vi "Parse_TCP_Message_From_Unity.vi"(5 "Tokenized message string array":string[](array[string])) -> (2 "task Over Message Received Flag":bool, 3 "Desired tensions by motor":T1, 4 "Control point position coords":dbl[](array[numeric]), 6 "Command string":string, 8 "Force field type specifier":string, 10 "Center point of FF":dbl[](array[numeric]), 13 "File information string":string, 14 "Trunk Structure Matrix":dbl[][](array[numeric]), 15 "Boundary points":dbl[](array[numeric]))   [LabVIEW 2024]
panel:
  out "Corresponding motor tensions":dbl[](array[numeric])
  out "Motor numbers":i32[](array[numeric])
  out "Most Recent Vicon Frame Number":u32
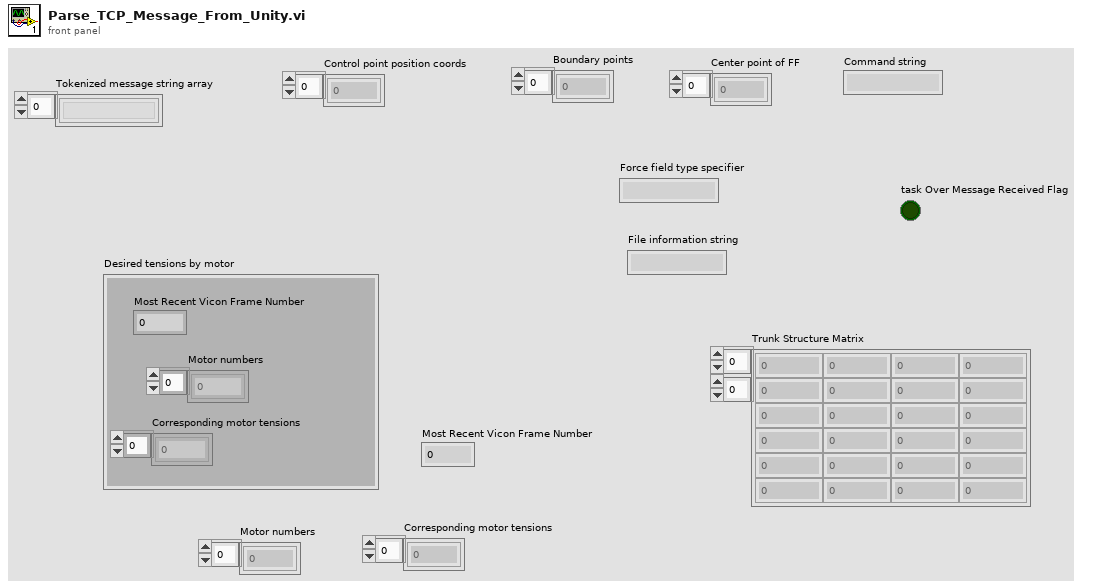
[diagram p1: front panel]
types:
  T1 = cluster{"Most Recent Vicon Frame Number":u32, "Corresponding motor tensions":dbl[], "Motor numbers":i32[]}
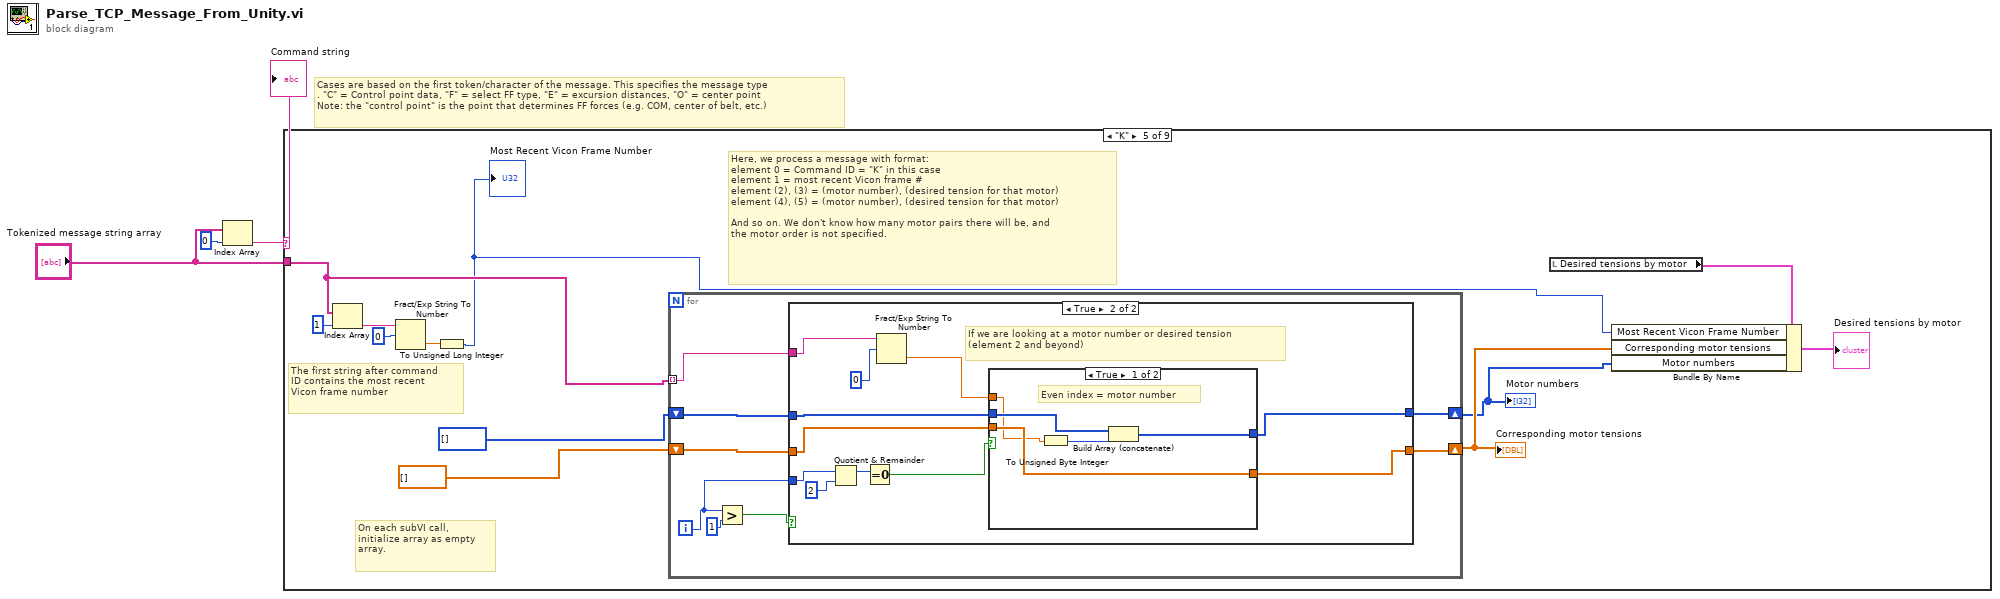
[diagram p0: block diagram]
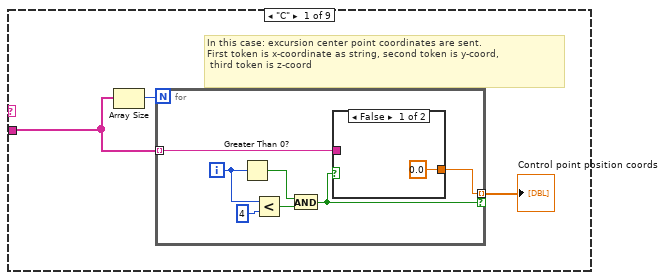
[diagram p2: hidden frame]
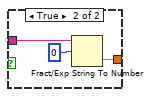
[diagram p3: hidden frame]
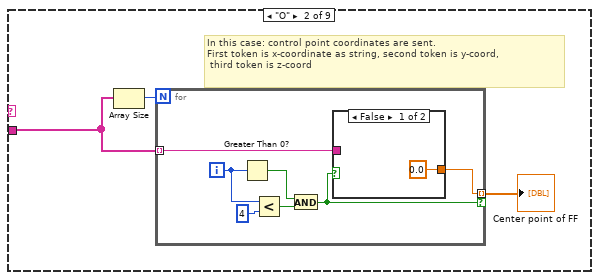
[diagram p4: hidden frame]
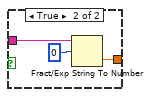
[diagram p5: hidden frame]
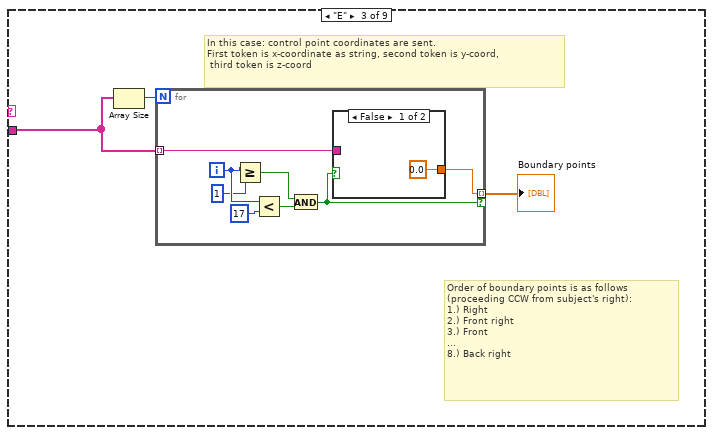
[diagram p6: hidden frame]
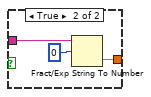
[diagram p7: hidden frame]
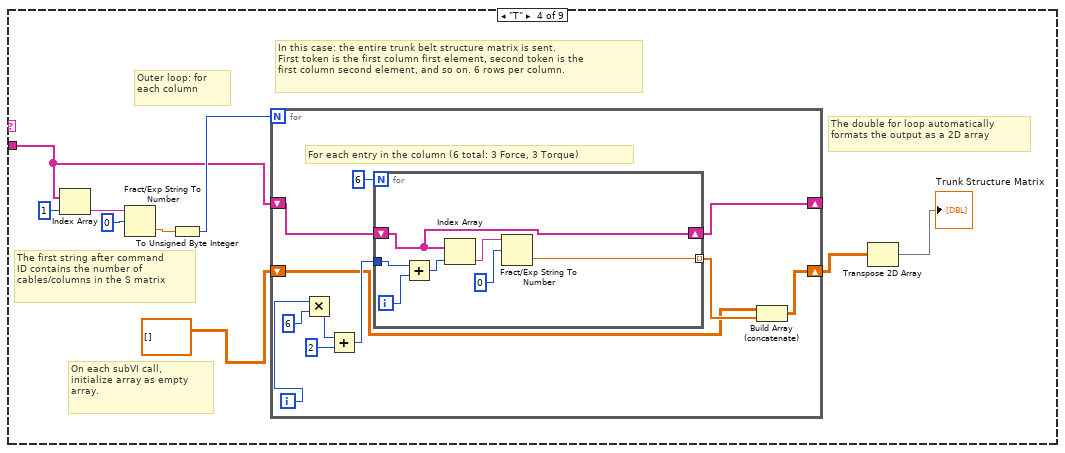
[diagram p8: hidden frame]
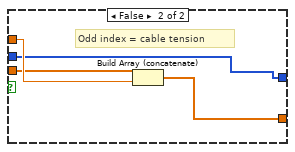
[diagram p10: hidden frame]
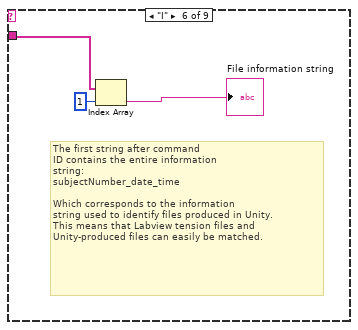
[diagram p11: hidden frame]
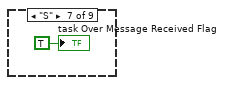
[diagram p12: hidden frame]
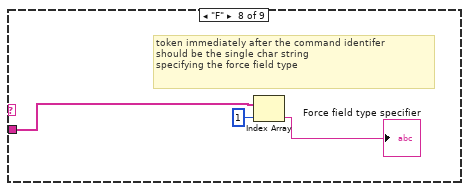
[diagram p13: hidden frame]
diagram:
  # "Cases are based on the first token/character of the message. This specifies the message type\n. \"C\" = Control point data, \"F\" = select FF type, \"E\" = excursion distances, \"O\" = center point \nNote: the \"control point\" is the point that determines FF forces (e.g. COM, center of belt, etc.)"
  n1 = Index Array(array="Tokenized message string array", index=0) -> (element=w2:string)
  "Command string" <- w2
  n2 = case shown="\"K\"" w2 {
    tunnel: "Tokenized message string array" -> [w4 w18 w32 w50 w82 w117 _ w121 _]
    frame "C" {
      # "In this case: excursion center point coordinates are sent. \nFirst token is x-coordinate as string, second token is y-coord,\n third token is z-coord"
      n3 = Array Size(array=w4) -> (size(s)=w6:i32)
      n4 = for {
        N: w6 -> [_]
        tunnel: w4 -> [w13] mode=indexing
        tunnel: [w12] -> w5 mode=indexing if=w7
        i -> [w9]
        n5 = Greater Than 0?(x=w9) -> (x > 0?=w11:bool)
        n6 = Less?(x=w9, y=4) -> (x < y?=w10:bool)
        n7 = And(x=w11, y=w10) -> (x .and. y?=w7:bool)
        n8 = case shown="False" w7 {
          tunnel: w13 -> [_ w17]
          tunnel: [0.0 w15] -> w12
          frame False {
          }
          frame True {
            n9 = Fract/Exp String To Number(string=w17, offset=0) -> (number=w15:dbl)  [unwired: 2 in, 1 out]
          }
        }
      }
      "Control point position coords" <- w5
    }
    frame "O" {
      # "In this case: control point coordinates are sent. \nFirst token is x-coordinate as string, second token is y-coord,\n third token is z-coord"
      n10 = Array Size(array=w18) -> (size(s)=w20:i32)
      n11 = for {
        N: w20 -> [_]
        tunnel: w18 -> [w27] mode=indexing
        tunnel: [w26] -> w19 mode=indexing if=w21
        i -> [w23]
        n12 = Greater Than 0?(x=w23) -> (x > 0?=w25:bool)
        n13 = Less?(x=w23, y=4) -> (x < y?=w24:bool)
        n14 = And(x=w25, y=w24) -> (x .and. y?=w21:bool)
        n15 = case shown="False" w21 {
          tunnel: w27 -> [_ w31]
          tunnel: [0.0 w29] -> w26
          frame False {
          }
          frame True {
            n16 = Fract/Exp String To Number(string=w31, offset=0) -> (number=w29:dbl)  [unwired: 2 in, 1 out]
          }
        }
      }
      "Center point of FF" <- w19
    }
    frame "E" {
      # "Order of boundary points is as follows \n(proceeding CCW from subject's right):\n1.) Right  \n2.) Front right\n3.) Front\n...\n8.) Back right"
      # "In this case: control point coordinates are sent. \nFirst token is x-coordinate as string, second token is y-coord,\n third token is z-coord"
      n17 = Array Size(array=w32) -> (size(s)=w34:i32)
      n18 = for {
        N: w34 -> [_]
        tunnel: w32 -> [w42] mode=indexing
        tunnel: [w41] -> w33 mode=indexing if=w38
        i -> [w37]
        n19 = Greater Or Equal?(x=w37, y=1) -> (x >= y?=w35:bool)
        n20 = Less?(x=w37, y=17) -> (x < y?=w40:bool)
        n21 = And(x=w35, y=w40) -> (x .and. y?=w38:bool)
        n22 = case shown="False" w38 {
          tunnel: w42 -> [_ w46]
          tunnel: [0.0 w44] -> w41
          frame False {
          }
          frame True {
            n23 = Fract/Exp String To Number(string=w46, offset=0) -> (number=w44:dbl)  [unwired: 2 in, 1 out]
          }
        }
      }
      "Boundary points" <- w33
    }
    frame "T" {
      # "On each subVI call,\ninitialize array as empty \narray."
      # "The double for loop automatically\nformats the output as a 2D array"
      # "Outer loop: for \neach column"
      # "The first string after command\nID contains the number of \ncables/columns in the S matrix"
      # "In this case: the entire trunk belt structure matrix is sent.\nFirst token is the first column first element, second token is the\nfirst column second element, and so on. 6 rows per column."
      n24 = Index Array(array=w50, index=1) -> (element=w54:string)
      n25 = Fract/Exp String To Number(string=w54, offset=0) -> (number=w52:dbl)  [unwired: 2 in, 1 out]
      n26 = To Unsigned Byte Integer(number=w52) -> (unsigned 8bit integer=w51:u8)
      n27 = for {
        N: w51 -> [_]
        shift-right: [w59] -> _
        shift-left: w50 -> [w65]
        shift-right: [w56] -> w49
        shift-left: dbl[][] [] -> [w57]
        i -> [w61]
        # "For each entry in the column (6 total: 3 Force, 3 Torque)"
        n28 = Multiply(x=w61, y=6) -> (x*y=w63:i32)
        n29 = Add(x=w63, y=2) -> (x+y=w62:i32)
        n30 = for {
          N: 6 -> [_]
          tunnel: w62 -> [w73]
          shift-right: [w67] -> w59
          shift-left: w65 -> [w67]
          tunnel: [w68] -> w58 mode=indexing
          i -> [w72]
          n31 = Add(x=w73, y=w72) -> (x+y=w71:i32)
          n32 = Index Array(array=w67, index=w71) -> (element=w70:string)
          n33 = Fract/Exp String To Number(string=w70, offset=0) -> (number=w68:dbl)  [unwired: 2 in, 1 out]
        }
        n34 = Build Array (concatenate)(w57, w58) -> (w56:dbl[][])
      }
      n35 = Transpose 2D Array(2D array=w49) -> (transposed array=→"Trunk Structure Matrix":dbl[][])
    }
    frame "K" {
      # "Here, we process a message with format: \nelement 0 = Command ID = \"K\" in this case\nelement 1 = most recent Vicon frame #\nelement (2), (3) = (motor number), (desired tension for that motor)\nelement (4), (5) = (motor number), (desired tension for that motor)\n\nAnd so on. We don't know how many motor pairs there will be, and \nthe motor order is not specified."
      # "On each subVI call,\ninitialize array as empty \narray."
      # "The first string after command\nID contains the most recent \nVicon frame number"
      n36 = Index Array(array=w82, index=1) -> (element=w84:string)
      n37 = Fract/Exp String To Number(string=w84, offset=0) -> (number=w75:dbl)  [unwired: 2 in, 1 out]
      n38 = To Unsigned Long Integer(number=w75) -> (unsigned 32bit integer=w74:u32)
      "Most Recent Vicon Frame Number" <- w74
      n39 = for {
        tunnel: w82 -> [w88] mode=indexing
        shift-right: [w87] -> w76
        shift-left: i32[] [] -> [w90]
        shift-right: [w86] -> w80
        shift-left: dbl[] [] -> [w89]
        i -> [w91]
        n40 = Greater?(x=w91, y=1) -> (0:w92:bool)
        n41 = case shown="True" w92 {
          tunnel: w91 -> [_ w106]
          tunnel: w90 -> [w95 w102]
          tunnel: w89 -> [w94 w101]
          tunnel: w88 -> [_ w99]
          tunnel: [w95 w97] -> w87
          tunnel: [w94 w96] -> w86
          frame False {
          }
          frame True {
            # "If we are looking at a motor number or desired tension \n(element 2 and beyond)"
            n42 = Quotient & Remainder(x=w106, y=2) -> (x-y*floor(x/y)=w104:i32)  [unwired: 1 out]
            n43 = Equal To 0?(x=w104) -> (x = 0?=w103:bool)
            n44 = Fract/Exp String To Number(string=w99, offset=0) -> (number=w98:dbl)  [unwired: 2 in, 1 out]
            n45 = case shown="True" w103 {
              tunnel: w102 -> [w111 w112]
              tunnel: w101 -> [w109 w114]
              tunnel: w98 -> [w108 w115]
              tunnel: [w110 w112] -> w97
              tunnel: [w109 w113] -> w96
              frame True {
                # "Even index = motor number"
                n46 = To Unsigned Byte Integer(number=w108) -> (unsigned 8bit integer=w107:u8)
                n47 = Build Array (concatenate)(w111, w107) -> (w110:i32[])
              }
              frame False {
                # "Odd index = cable tension"
                n48 = Build Array (concatenate)(w114, w115) -> (w113:dbl[])
              }
            }
          }
        }
      }
      "Corresponding motor tensions" <- w80
      "Motor numbers" <- w76
      n49 = local read "Desired tensions by motor"() -> (w81:T1)
      n50 = Bundle By Name(cluster=w81, "Most Recent Vicon Frame Number"=w74, "Corresponding motor tensions"=w80, "Motor numbers"=w76) -> (→"Desired tensions by motor":T1)
    }
    frame "I" {
      # "The first string after command\nID contains the entire information\nstring:\nsubjectNumber_date_time \n\nWhich corresponds to the information\nstring used to identify files produced in Unity. \nThis means that Labview tension files and \nUnity-produced files can easily be matched."
      n51 = Index Array(array=w117, index=1) -> (element=→"File information string":string)
    }
    frame "S" {
      "task Over Message Received Flag" <- TRUE ("task Over Message Received Flag")
    }
    frame "F" {
      # "token immediately after the command identifer \nshould be the single char string\nspecifying the force field type"
      n52 = Index Array(array=w121, index=1) -> (element=→"Force field type specifier":string)
    }
    frame "Unknown command type", Default {
    }
  }
